vi "Get Name.vi"(11 "logger in":refnum<class "Logger.lvclass">) -> (2 "name":string, 3 "logger out":refnum<class "Logger.lvclass">)   [LabVIEW 2018, in "Logging.lvlib" / "Logger.lvclass"]
uses:
  Logger.lvclass
  Logger.lvclass/Logger.ctl
panel:
  # "Connector Pane"
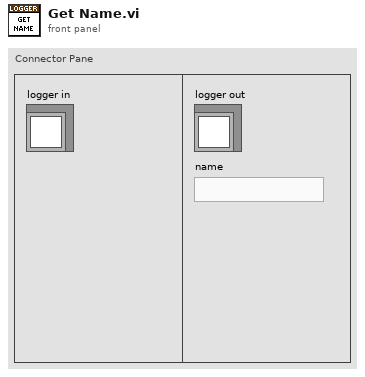
[diagram p1: front panel]
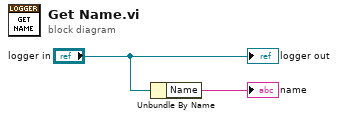
[diagram p0: block diagram]
diagram:
  n1 = Unbundle By Name("logger in") -> ("Name"=→"name":string)
  "logger out" <- "logger in"
